vi "Sequence.vi"   [LabVIEW 2023]
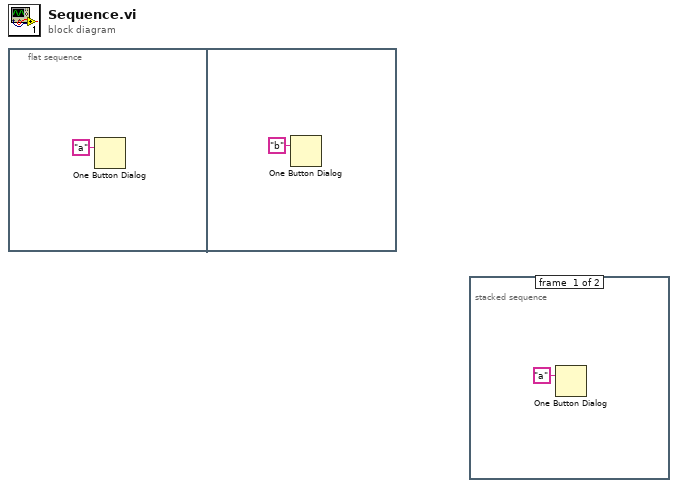
[diagram p0: block diagram]
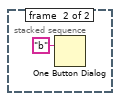
[diagram p2: hidden frame]
diagram:
  n1 = flat-sequence {
    frame #0 {
      n2 = One Button Dialog(message="a") -> ()  [unwired: 1 in, 1 out]
    }
    frame #1 {
      n3 = One Button Dialog(message="b") -> ()  [unwired: 1 in, 1 out]
    }
  }
  n4 = stacked-sequence {
    frame #0 {
      n5 = One Button Dialog(message="a") -> ()  [unwired: 1 in, 1 out]
    }
    frame #1 {
      n6 = One Button Dialog(message="b") -> ()  [unwired: 1 in, 1 out]
    }
  }
